vi "Goto Wavelength.vi"(8 "error in (no error)":errorcluster, 10 "WAVELENGTH":dbl[unit] min=0.0 max=0.016777215000000012 step=1.0000000000000007e-11 format="%.2f", 11 "VISA resource name":refnum<visa-resource-name>) -> (0 "error out":errorcluster, 3 "VISA resource name out":refnum<visa-resource-name>)   [LabVIEW 2015, in "Digikrom DK24x.lvlib"]
doc: "This command moves the monochromator to a selected position. Valid values of position depend on the gratings installed in the instrument."
uses:
  Digikrom DK24x.lvlib
  Private/Command.ctl
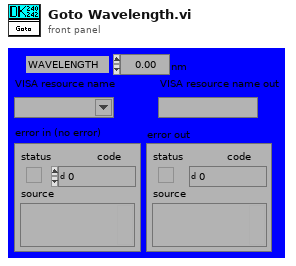
[diagram p1: front panel]
types:
  T1 = typedef "Digikrom DK24x.lvlib/Command.ctl" = u8
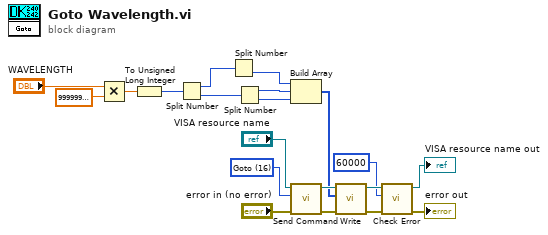
[diagram p0: block diagram]
diagram:
  w1 = T1 16 items=["Cancel"=24, "Clear"=25, "CSR"=28, "Echo"=27, "Filter"=15, "Gcal"=18, "Goto"=16, "Grtid?"=19, "Grtsel"=26, "NOVRAM Read"=56, "NOVRAM Write"=59, "Reset"=255, "Scan"=12, "Scan Up"=9, "Scan Down"=3, "Serial?"=33, "Slew Up"=8, "Slew Down"=2, "Slit Reset"=43, "Slit?"=30, "Sltadj"=14, "Speed"=13, "Sspeed?"=21, "Step Down"=1, "Step Up"=7, "S1adj"=31, "S2adj"=32, "S3adj"=34, "S1cal"=22, "S2cal"=23, "S3cal"=35, "Test"=17, "Type"=57, "Wave?"=29, "Zero"=52] ("Command")
  n1 = Multiply(x="WAVELENGTH", y=dbl[unit] 99999999999.99992 ("/nm")) -> (x*y=w12:dbl)
  n2 = To Unsigned Long Integer(number=w12) -> (unsigned 32bit integer=w17:u32)
  n3 = Split Number(x=w17) -> (hi(x)=w18:u16, lo(x)=w19:u16)
  n4 = Split Number(x=w18) -> (lo(x)=w16:u8)  [unwired: 1 out]
  n5 = Split Number(x=w19) -> (hi(x)=w15:u8, lo(x)=w14:u8)
  n6 = Build Array(w16, w15, w14) -> (w2:u8[])
  n7 = call "Send Command.vi"("error in (no error)"="error in (no error)", "Command"=w1, "VISA resource name"="VISA resource name") -> ("error out"=w6:errorcluster, "VISA resource name out"=w5:refnum<visa-resource-name>)  [unwired: 7 out]
  n8 = call "Write.vi"("error in (no error)"=w6, "Byte Array"=w2, "VISA resource name"=w5) -> ("error out"=w9:errorcluster, "VISA resource name out"=w8:refnum<visa-resource-name>)  [unwired: 7 out]
  n9 = call "Check Error.vi"("error in"=w9, "timeout"=60000, "VISA resource name in"=w8) -> ("error out"=→"error out":errorcluster, "VISA resource name out"=→"VISA resource name out":refnum<visa-resource-name>)  [unwired: 7 out]
